vi "Read Image delays.vi"(8 "error in (no error)":errorcluster, 11 "Header in":refnum<class "Header.lvclass">) -> (0 "error out":errorcluster, 2 "Image delays":string[](array[string]), 3 "Header out":refnum<class "Header.lvclass">)   [LabVIEW 2018, in "Header.lvclass"]
uses:
  Header.lvclass
  C:/Users/observer/Desktop/SPARC4_ACS/Simulated_Header/Simulated_Header.lvclass
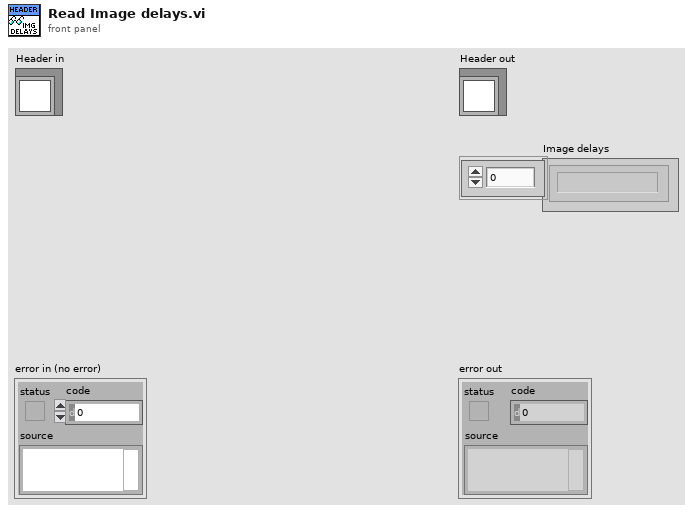
[diagram p1: front panel]
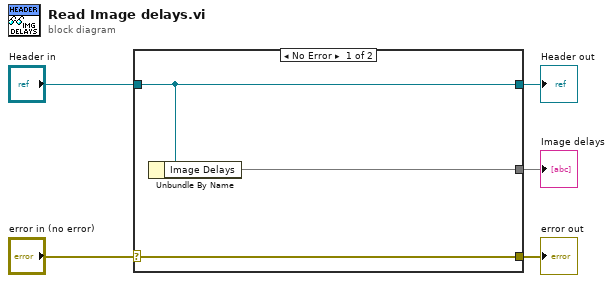
[diagram p0: block diagram]
diagram:
  n1 = case shown="No Error" "error in (no error)" {
    selector: "error in (no error)" -> [w8 w9]
    tunnel: [w8 w9] -> w4
    tunnel: [w7 w10] -> w2
    tunnel: "Header in" -> [w7 w10]
    tunnel: [w6 _] -> w1
    frame No Error {
      n2 = Unbundle By Name(w7) -> ("Image Delays"=w6)
    }
    frame Error {
    }
  }
  "error out" <- w4
  "Header out" <- w2
  "Image delays" <- w1
